vi "GetBooleanReference.vi"(8 "error in":errorcluster, 11 "Boolean in":refnum<class "Boolean.lvclass">) -> (0 "error out":errorcluster, 1 "Boolean reference":refnum<vi>, 3 "Boolean out":refnum<class "Boolean.lvclass">)   [LabVIEW 2014, in "Boolean.lvclass"]
uses:
  Boolean.lvclass
  Generic/Generic.lvclass
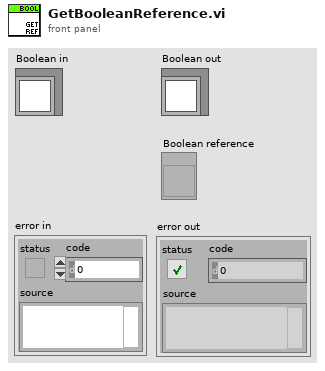
[diagram p1: front panel]
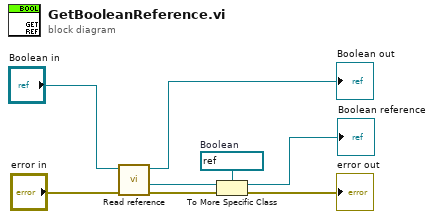
[diagram p0: block diagram]
diagram:
  w8 = refnum<vi> refnum  # Boolean
  n1 = call "Read reference.vi"("error in"="error in", "GObject in"="Boolean in") -> ("error out"=w7:errorcluster, "reference"=w6:refnum<vi>, "GObject out"=→"Boolean out":refnum<class "Boolean.lvclass">)  [unwired: 5 in]
  n2 = To More Specific Class(target class=w8, reference=w6, error in=w7) -> (specific class reference=→"Boolean reference":refnum<vi>, error out=→"error out":errorcluster)
